vi "Manipulate_Pops.vi"(7 "Target array":dbl[](array[numeric]), 8 "Relaxation Rate":dbl, 9 "Microwave Power":dbl, 10 "RF Array":dbl[](array[numeric]), 11 "Pop Array":dbl[](array[numeric])) -> (3 "Decayed/Grown Array":dbl[](array[numeric]))   [LabVIEW 2018]
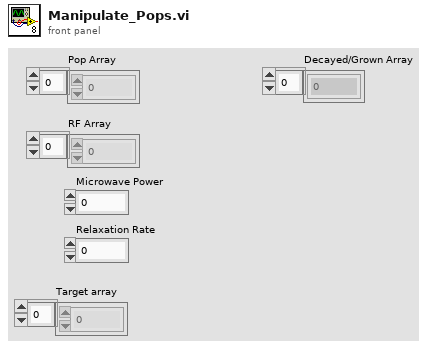
[diagram p1: front panel]
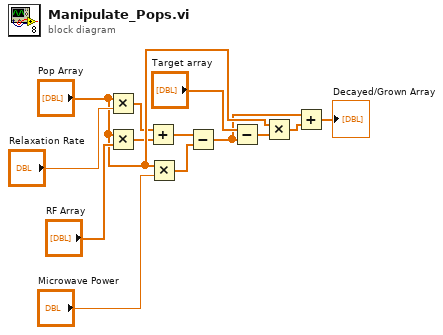
[diagram p0: block diagram]
diagram:
  n1 = Multiply(x="Pop Array", y="Relaxation Rate") -> (x*y=w8:dbl[])
  n2 = Multiply(x="Pop Array", y="RF Array") -> (x*y=w9:dbl[])
  n3 = Add(x=w8, y=w9) -> (x+y=w7:dbl[])
  n4 = Multiply(x="Pop Array", y="Microwave Power") -> (x*y=w6:dbl[])
  n5 = Subtract(x=w7, y=w6) -> (x-y=w1:dbl[])
  n6 = Subtract(x="Target array", y=w1) -> (x-y=w3:dbl[])
  n7 = Multiply(x="Pop Array", y=w3) -> (x*y=w5:dbl[])
  n8 = Add(x=w1, y=w5) -> (x+y=→"Decayed/Grown Array":dbl[])
